vi "Configure Feed Manager Feeds.vi"(8 "error in (no error)":errorcluster, 11 "feeds INI Filepath":path) -> (0 "error out":errorcluster, 2 "cancelled":bool)   [LabVIEW 2014]
doc: "Launches the Configure Feeds window, which allows the user to create, add, and remove feeds for the NIPM Feed Manager to manage."
uses:
  Configure Feeds States.ctl
  Configure Feeds State Data.ctl
  <vilib>/Utility/config.llb/Write Key (String).vi
  <vilib>/Utility/config.llb/NI_LVConfig.lvlib
panel:
  in  "Cancel Button":bool
  in  "OK Button":bool
  in  "Remove Feed":bool
  in  "Add Feed":bool
  in  "Configured Feeds":i32(listbox)
  # "The Feed Manager utility is currently managing the following feeds:"
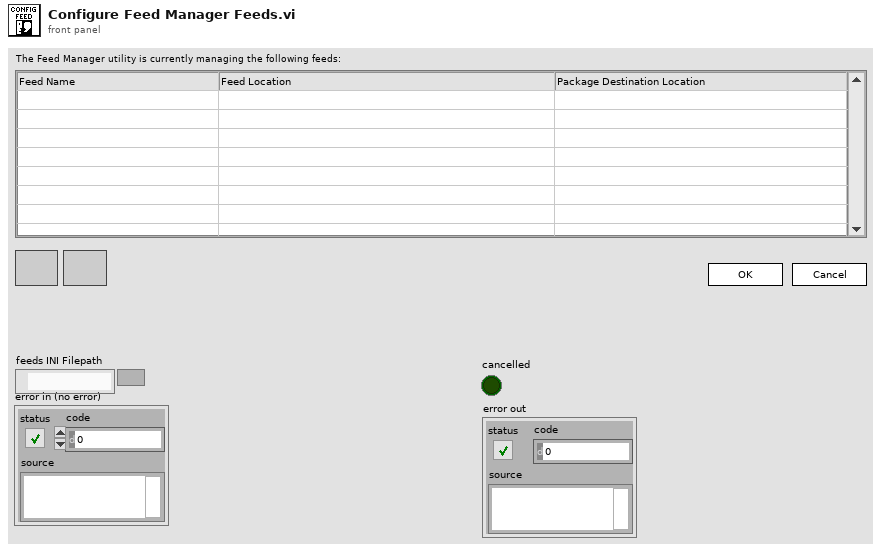
[diagram p1: front panel]
types:
  T1 = typedef "Configure Feeds State Data.ctl" = cluster{"Configured Feeds":string[][], "Selected Feed":i32, "Feeds INI Filepath":path}
  T2 = typedef "Configure Feeds States.ctl" = enum16{"Initialize", "Display Configured Feeds", "Wait on Event", "Add Feed", "Remove Feed", "Update INI File", "Exit"}
  T3 = enum8{"Enabled", "Disabled", "Disabled and Grayed Out"}
  T4 = typedef "Feed Info.ctl" = cluster{"Feed Name":string, "Feed Folderpath":string, "Package Destination Folderpath":string}
  T5 = typedef "NI_LVConfig.lvlib/Config Data RefNum.ctl" = refnum<k1>
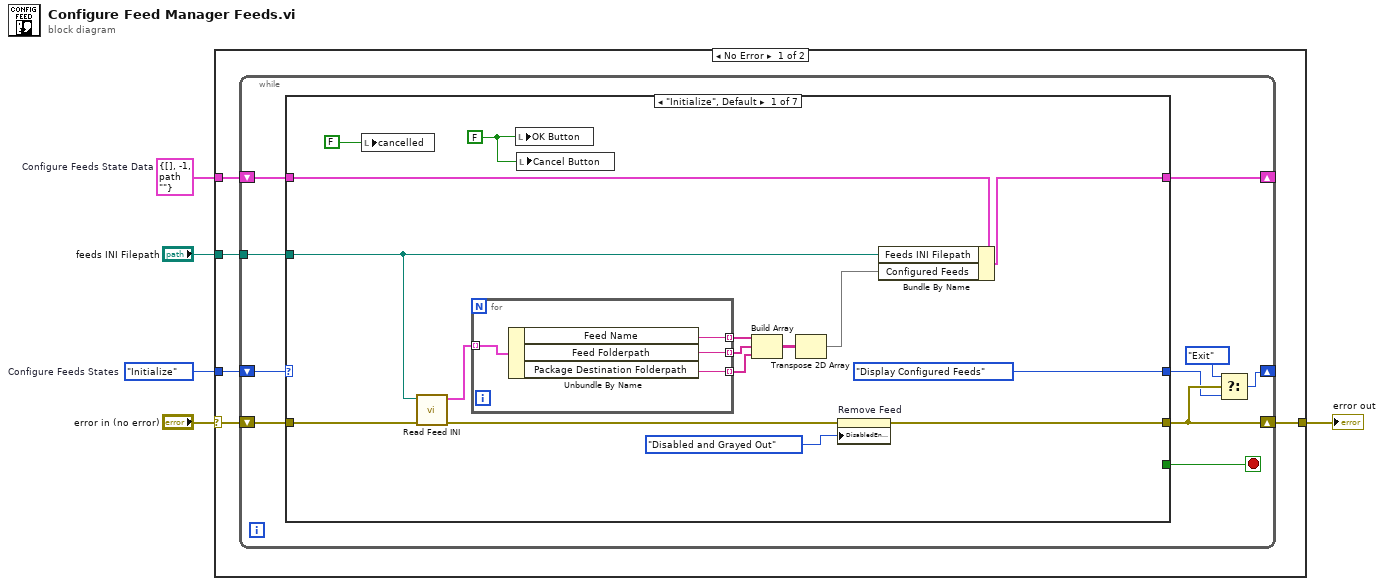
[diagram p0: block diagram]
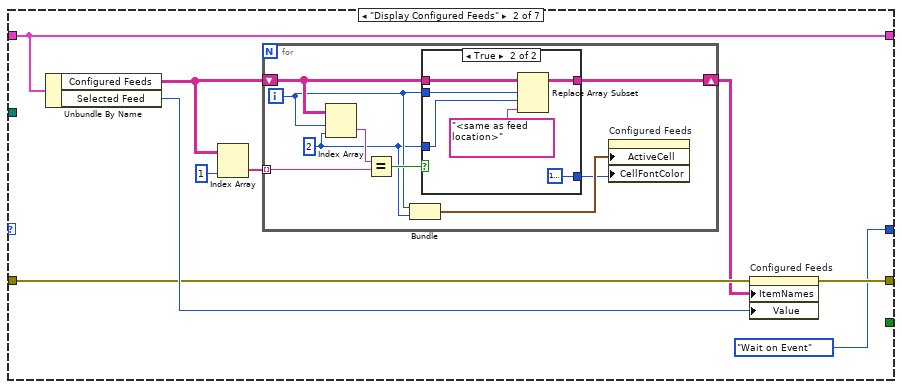
[diagram p2: hidden frame]
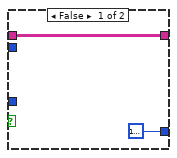
[diagram p3: hidden frame]
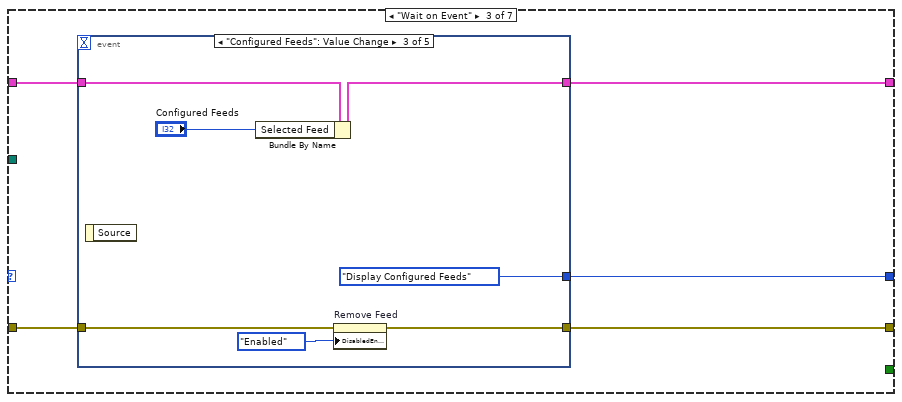
[diagram p4: hidden frame]
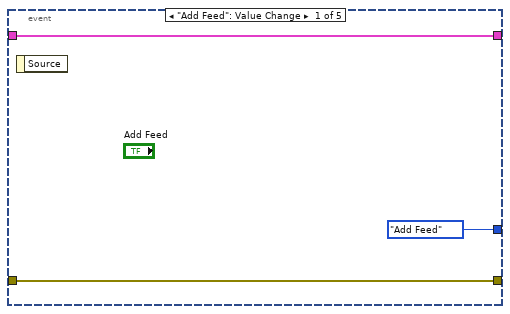
[diagram p5: hidden frame]
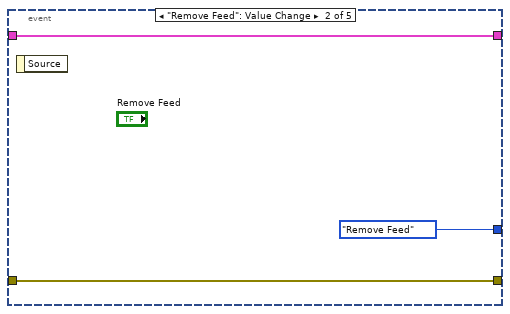
[diagram p6: hidden frame]
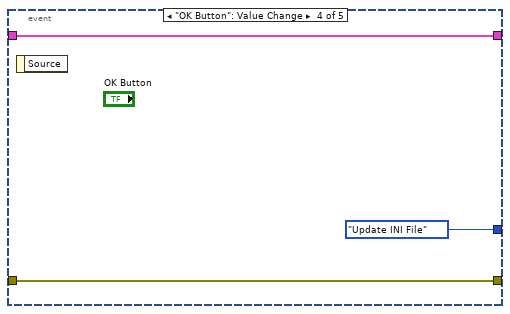
[diagram p7: hidden frame]
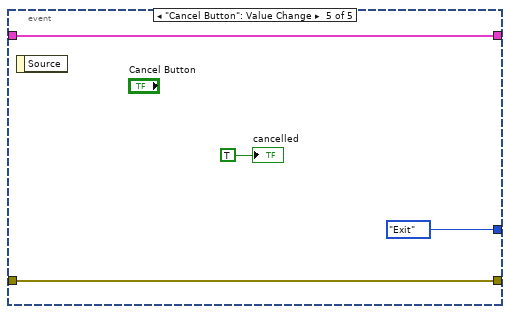
[diagram p8: hidden frame]
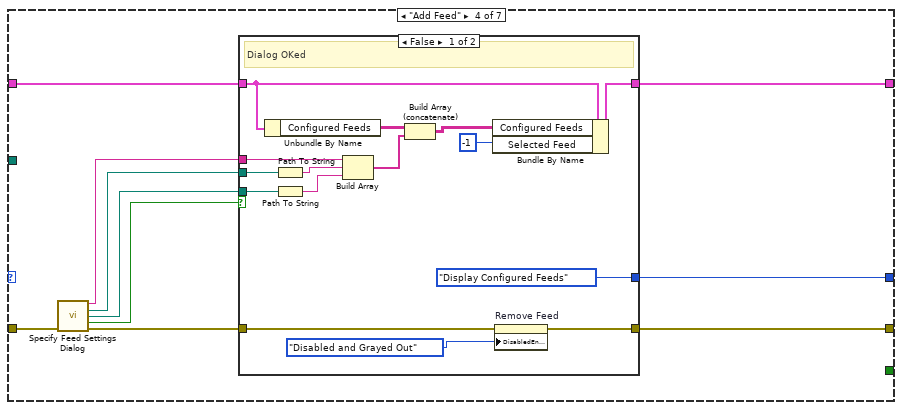
[diagram p9: hidden frame]
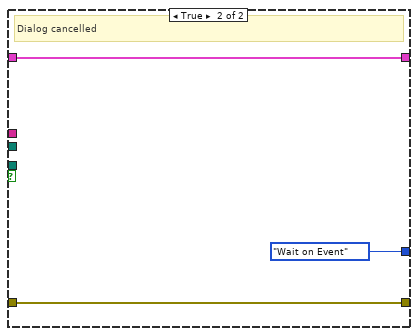
[diagram p10: hidden frame]
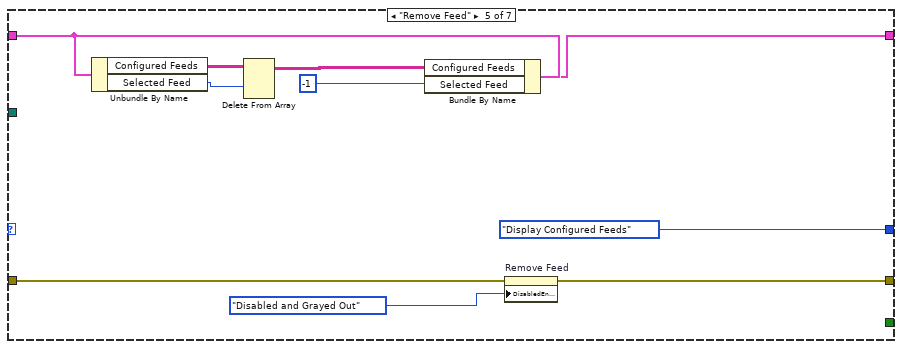
[diagram p11: hidden frame]
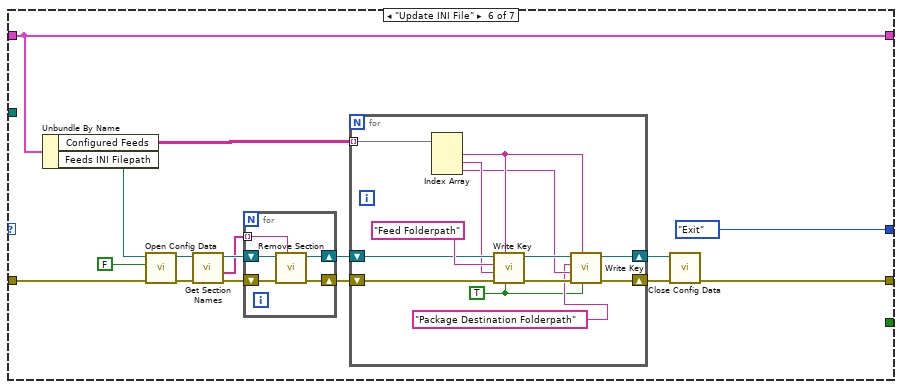
[diagram p12: hidden frame]
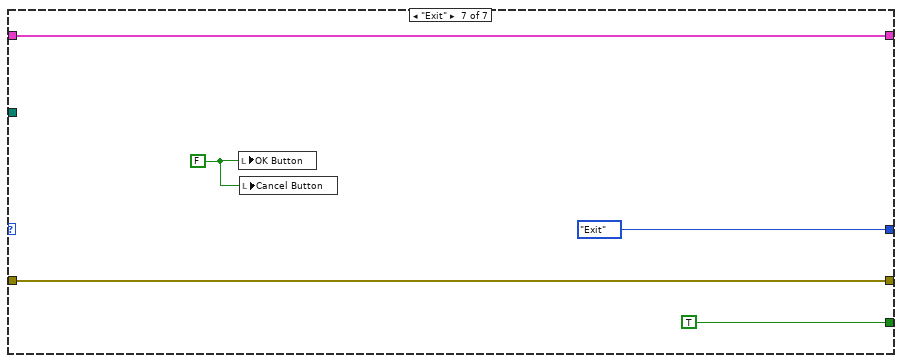
[diagram p13: hidden frame]
diagram:
  w4 = T1 {"Configured Feeds"=[], "Selected Feed"=-1, "Feeds INI Filepath"=path ""}  # Configure Feeds State Data
  w5 = Configure_Feeds_States."Initialize"  # Configure Feeds States
  n1 = case shown="No Error" "error in (no error)" {
    selector: "error in (no error)" -> [w6 w169]
    tunnel: w5 -> [w10 _]
    tunnel: w4 -> [w9 _]
    tunnel: [w8 w169] -> w3
    tunnel: "feeds INI Filepath" -> [w7 _]
    frame No Error {
      n2 = while {
        shift-right: [w13] -> _
        shift-left: w10 -> [w20]
        shift-right: [w18] -> _
        shift-left: w9 -> [w19]
        shift-right: [w15] -> w8
        shift-left: w6 -> [w17]
        tunnel: w7 -> [w11]
        stop <- w16 stop-if-true
        n3 = case shown="\"Initialize\", Default" w20 {
          tunnel: w19 -> [w36 w48 w70 w99 w128 w140 w168]
          tunnel: [w35 w48 w69 w98 w127 w140 w168] -> w18
          tunnel: [Configure_Feeds_States."Display Configured Feeds" ("Configure Feeds States") Configure_Feeds_States."Wait on Event" ("Configure Feeds States") w71 w93 Configure_Feeds_States."Display Configured Feeds" ("Configure Feeds States") Configure_Feeds_States."Exit" ("Configure Feeds States") Configure_Feeds_States."Exit" ("Configure Feeds States")] -> w14
          tunnel: w17 -> [w29 w46 w68 w101 w121 w145 w167]
          tunnel: [w25 w49 w67 w94 w120 w131 w167] -> w15
          tunnel: [_ _ _ _ _ _ TRUE] -> w16
          tunnel: w11 -> [w21 _ _ _ _ _ _]
          frame "Initialize", Default {
            w22 = FALSE
            n4 = local write "cancelled"(FALSE ("cancelled")) -> ()
            n5 = call "Read Feed INI.vi"("error in (no error)"=w29, "feeds INI filepath"=w21) -> ("error out"=w26:errorcluster, "Feeds"=w30:T4[])  [unwired: 8 in]
            n6 = for {
              tunnel: w30 -> [w40] mode=indexing
              tunnel: [w39] -> w31 mode=indexing
              tunnel: [w38] -> w32 mode=indexing
              tunnel: [w37] -> w23 mode=indexing
              n7 = Unbundle By Name(w40) -> ("Feed Name"=w39:string, "Feed Folderpath"=w38:string, "Package Destination Folderpath"=w37:string)
            }
            n8 = local write "OK Button"(w22) -> ()
            n9 = local write "Cancel Button"(w22) -> ()
            n10 = Build Array(w31, w32, w23) -> (w33:string[][])
            n11 = Transpose 2D Array(2D array=w33) -> (transposed array=w28:string[][])
            n12 = property on="Remove Feed" class="Bool"(error in=w26, "DisabledEnum"=T3."Disabled and Grayed Out" ("Disabled")) -> (error out=w25:errorcluster)  [unwired: 1 in, 1 out]
            n13 = Bundle By Name(cluster=w36, "Feeds INI Filepath"=w21, "Configured Feeds"=w28) -> (w35:T1)
          }
          frame "Display Configured Feeds" {
            n14 = Unbundle By Name(w48) -> ("Configured Feeds"=w42:string[][], "Selected Feed"=w47:i32)
            n15 = Index Array(array=w42, index (col)=1 ("disabled index (col)")) -> (element=w43:string[])  [unwired: 1 in]
            n16 = for {
              tunnel: w43 -> [w57] mode=indexing
              shift-right: [w54] -> w41
              shift-left: w42 -> [w56]
              i -> [w53]
              w52 = 2 ("disabled index (col)")
              n17 = Index Array(array=w56, index (row)=w53, index (col)=w52) -> (element=w58:string)
              n18 = Equal?(x=w58, y=w57) -> (x = y?=w55:bool)
              n19 = Bundle(w53, "disabled index (col)"=w52) -> (w51:cluster{i32, "disabled index (col)":i32})  [unwired: 1 in]
              n20 = case shown="True" w55 {
                tunnel: w56 -> [w60 w66]
                tunnel: [w60 w65] -> w54
                tunnel: w53 -> [_ w63]
                tunnel: w52 -> [_ w62]
                tunnel: [u32 16777222 u32 16777238] -> w50
                frame False {
                }
                frame True {
                  n21 = Replace Array Subset(array=w66, new element="<same as feed location>" ("new element/subarray"), index (row)=w63, index (col)=w62) -> (w65:string[][])
                }
              }
              n22 = property on="Configured Feeds" class="MCListbox (strict)"("ActiveCell"=w51, "CellFontColor"=w50) -> ()  [unwired: 2 in, 2 out]
            }
            n23 = property on="Configured Feeds" class="MCListbox (strict)"(error in=w46, "ItemNames"=w41, "Value"=w47) -> (error out=w49:errorcluster)  [unwired: 1 in, 1 out]
          }
          frame "Wait on Event" {
            n24 = event shown="[2] \"Configured Feeds\": Value Change" {
              selector: _ -> [_ _ _ _ _]
              dyn-events: _ -> [_ _ _ _ _]
              timeout: _ -> [_ _ _ _ _]
              tunnel: [Configure_Feeds_States."Add Feed" ("Configure Feeds States") Configure_Feeds_States."Remove Feed" ("Configure Feeds States") Configure_Feeds_States."Display Configured Feeds" ("Configure Feeds States") Configure_Feeds_States."Update INI File" ("Configure Feeds States") Configure_Feeds_States."Exit" ("Configure Feeds States")] -> w71
              tunnel: w70 -> [w73 w76 w83 w87 w91]
              tunnel: [w73 w76 w82 w87 w91] -> w69
              tunnel: w68 -> [w72 w75 w79 w86 w90]
              tunnel: [w72 w75 w78 w86 w90] -> w67
              event "Add Feed": Value Change {
                n25 = event-data() -> ()  [unwired: 1 in, 1 out]
              }
              event "Remove Feed": Value Change {
                n26 = event-data() -> ()  [unwired: 1 in, 1 out]
              }
              event "Configured Feeds": Value Change {
                n27 = event-data() -> ()  [unwired: 1 in, 1 out]
                n28 = Bundle By Name(cluster=w83, "Selected Feed"="Configured Feeds") -> (w82:T1)
                n29 = property on="Remove Feed" class="Bool"(error in=w79, "DisabledEnum"=T3."Enabled" ("Disabled")) -> (error out=w78:errorcluster)  [unwired: 1 in, 1 out]
              }
              event "OK Button": Value Change {
                n30 = event-data() -> ()  [unwired: 1 in, 1 out]
              }
              event "Cancel Button": Value Change {
                n31 = event-data() -> ()  [unwired: 1 in, 1 out]
                "cancelled" <- TRUE ("cancelled")
              }
            }
          }
          frame "Add Feed" {
            n32 = call "Specify Feed Settings Dialog.vi"("error in (no error)"=w101) -> ("feed name out"=w97:string, "feed folderpath out"=w96:path, "package destination folderpath out"=w92:path, "cancelled?"=w100:bool, "error out"=w95:errorcluster)  [unwired: 10 in]
            n33 = case shown="False" w100 {
              tunnel: w99 -> [w115 w119]
              tunnel: [w116 w119] -> w98
              tunnel: w97 -> [w112 _]
              tunnel: w96 -> [w113 _]
              tunnel: w95 -> [w105 w118]
              tunnel: [w104 w118] -> w94
              tunnel: [Configure_Feeds_States."Display Configured Feeds" ("Configure Feeds States") Configure_Feeds_States."Wait on Event" ("Configure Feeds States")] -> w93
              tunnel: w92 -> [w103 _]
              frame False {
                # "Dialog OKed"
                n34 = Unbundle By Name(w115) -> ("Configured Feeds"=w114:string[][])
                n35 = Path To String(path=w113) -> (string=w111:string)
                n36 = Path To String(path=w103) -> (string=w102:string)
                n37 = Build Array(w112, w111, w102) -> (w110:string[])
                n38 = Build Array (concatenate)(w114, w110) -> (w109:string[][])
                n39 = Bundle By Name(cluster=w115, "Configured Feeds"=w109, "Selected Feed"=-1) -> (w116:T1)
                n40 = property on="Remove Feed" class="Bool"(error in=w105, "DisabledEnum"=T3."Disabled and Grayed Out" ("Disabled")) -> (error out=w104:errorcluster)  [unwired: 1 in, 1 out]
              }
              frame True {
                # "Dialog cancelled"
              }
            }
          }
          frame "Remove Feed" {
            n41 = Unbundle By Name(w128) -> ("Configured Feeds"=w126:string[][], "Selected Feed"=w125:i32)
            n42 = Delete From Array(array=w126, index (row)=w125) -> (array with subset deleted=w124:string[][])  [unwired: 2 in, 1 out]
            n43 = Bundle By Name(cluster=w128, "Configured Feeds"=w124, "Selected Feed"=-1) -> (w127:T1)
            n44 = property on="Remove Feed" class="Bool"(error in=w121, "DisabledEnum"=T3."Disabled and Grayed Out" ("Disabled")) -> (error out=w120:errorcluster)  [unwired: 1 in, 1 out]
          }
          frame "Update INI File" {
            n45 = Unbundle By Name(w140) -> ("Configured Feeds"=w133:string[][], "Feeds INI Filepath"=w139:path)
            n46 = call <vilib>:"Open Config Data.vi"("error in (no error)"=w145, "create file if necessary (T)"=FALSE, "configuration file path"=w139) -> ("error out"=w143:errorcluster, "refnum"=w141:T5)  [unwired: 6 in, 1 out]
            n47 = call <vilib>:"Get Section Names.vi"("error in (no error)"=w143, "refnum"=w141) -> ("error out"=w142:errorcluster, "section names"=w136:string[], "refnum out"=w137:T5)  [unwired: 7 in]
            n48 = for {
              shift-right: [w162] -> w135
              shift-left: w142 -> [w163]
              tunnel: w136 -> [w160] mode=indexing
              shift-right: [w159] -> w132
              shift-left: w137 -> [w161]
              n49 = call <vilib>:"Remove Section.vi"("section"=w160, "error in (no error)"=w163, "refnum"=w161) -> ("error out"=w162:errorcluster, "refnum out"=w159:T5)  [unwired: 6 in, 1 out]
            }
            n50 = for {
              shift-right: [w152] -> w134
              shift-left: w135 -> [w156]
              tunnel: w133 -> [w158] mode=indexing
              shift-right: [w150] -> w130
              shift-left: w132 -> [w154]
              w146 = TRUE ("write raw string? (F)")
              n51 = Index Array(array=w158) -> (element #1=w149:string, element #2=w153:string, element #3=w148:string)  [unwired: 3 in]
              n52 = call-poly <vilib>:"Write Key.vi"("write raw string? (F)"=w146, "section"=w149, "error in (no error)"=w156, "value"=w153, "key"="Feed Folderpath", "refnum"=w154) -> ("error out"=w157:errorcluster, "refnum out"=w151:T5)  [unwired: 3 in, 1 out]
              n53 = call-poly <vilib>:"Write Key.vi"("write raw string? (F)"=w146, "section"=w149, "error in (no error)"=w157, "value"=w148, "key"="Package Destination Folderpath", "refnum"=w151) -> ("error out"=w152:errorcluster, "refnum out"=w150:T5)  [unwired: 3 in, 1 out]
            }
            n54 = call <vilib>:"Close Config Data.vi"("error in (no error)"=w134, "refnum"=w130) -> ("error out"=w131:errorcluster)  [unwired: 8 in, 1 out]
          }
          frame "Exit" {
            w164 = FALSE
            n55 = local write "OK Button"(w164) -> ()
            n56 = local write "Cancel Button"(w164) -> ()
          }
        }
        n57 = Select(t=Configure_Feeds_States."Exit", s=w15, f=w14) -> (s? t:f=w13:T2)
      }
    }
    frame Error {
    }
  }
  "error out" <- w3
